vi "FP_Place FP on Point.vi"(8 "Error":errorcluster, 9 "FPSet":T1={"Menu Bar"=FALSE, "Position"=enum."MID-CTR", "Decoration index"=0, "border(px)"=-2, "Point"={"Left"=0, "Top"=0}}, 11 "VI Ref":refnum<vi>) -> (0 "Error Out":errorcluster, 3 "VI Ref Out":refnum<vi>)   [LabVIEW 2020]
doc: "sets up a fp to center of monitor 1 around largest decoration. shows scroll bars if developing and hides them if not."
uses:
  TypeDefs_Utility/Cluster_FP on Point Set.ctl
  TypeDefs_Utility/ENUM RB_Pos_Quadrant Position.ctl
  TypeDefs_Utility/Cluster_Top Left position.ctl
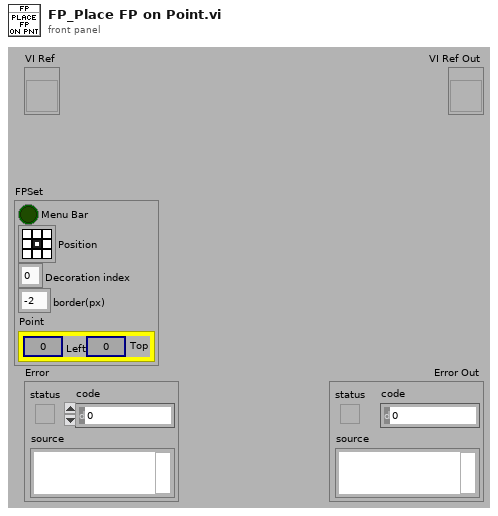
[diagram p1: front panel]
types:
  T1 = typedef "Cluster_FP on Point Set.ctl" = cluster{"Menu Bar":bool, "Position":T2, "Decoration index":i32, "border(px)":i32, "Point":T3}
  T2 = typedef "ENUM RB_Pos_Quadrant Position.ctl" = enum32{"LFT-TOP", "MID-TOP", "RGT-TOP", "LFT-CTR", "MID-CTR", "RGT-CTR", "LFT-BOT", "MID-BOT", "RGT-BOT"}
  T3 = typedef "Cluster_Top Left position.ctl" = cluster{"Left":i32, "Top":i32}
  T4 = enum32{"invalid app kind", "Development System", "Run Time System", "Student Edition", "Embedded LabVIEW", "Evaluation", "Custom"}
  T5 = enum32{"Invalid", "Standard", "Closed", "Hidden", "Minimized", "Maximized"}
  T6 = enum16{"Always On", "Always Off", "Off While Running"}
  T7 = typedef "LVRectTypeDef.ctl" = cluster{"Left":i16, "Top":i16, "Right":i16, "Bottom":i16}
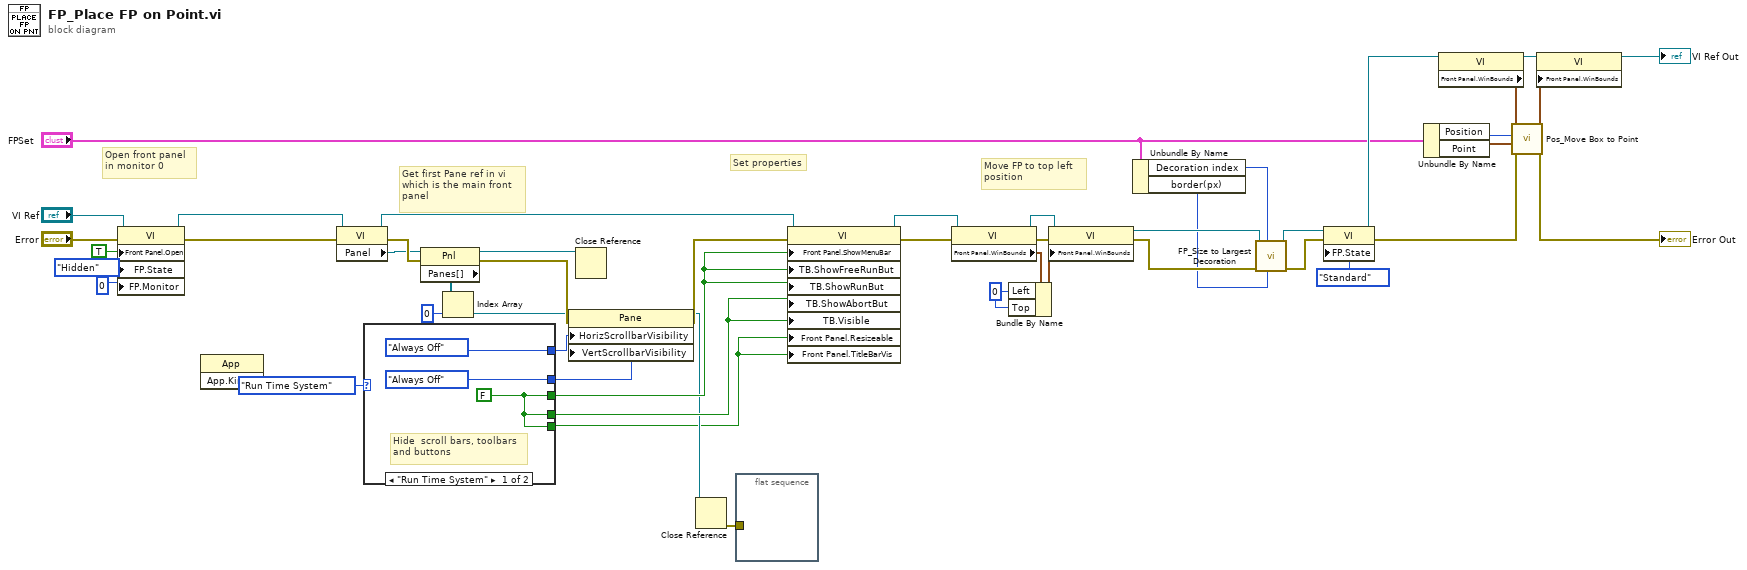
[diagram p0: block diagram]
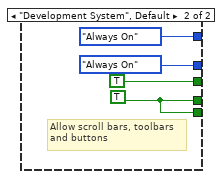
[diagram p2: hidden frame]
diagram:
  w24 = i16 0 ("left")
  # "Move FP to top left\nposition"
  # "Set properties"
  # "Get first Pane ref in vi\nwhich is the main front\npanel"
  # "Open front panel\nin monitor 0"
  n1 = property class="VI"(reference="VI Ref", error in="Error", "Front Panel.Open"=TRUE ("Front Panel Window:Open"), "FP.State"=T5."Hidden" ("Front Panel Window:State"), "FP.Monitor"=u16 0 ("Front Panel Window:Monitor")) -> (reference out=w19:refnum<vi>, error out=w20:errorcluster)
  n2 = property class="App" props=["App.Kind"]() -> ()  [unwired: 2 in, 3 out]
  n3 = property class="VI"(reference=w19, error in=w20) -> (reference out=w31:refnum<vi>, error out=w44:errorcluster, "Panel"=w40:refnum<vi>)
  n4 = case shown="\"Run Time System\"" T4."Run Time System" ("App.Kind") {
    tunnel: [T6."Always Off" ("Horizontal Scrollbar Visibility") T6."Always On" ("Horizontal Scrollbar Visibility")] -> w46
    tunnel: [w49 TRUE ("Front Panel Window:Show Menu Bar")] -> w11
    tunnel: [w49 w52] -> w33
    tunnel: [T6."Always Off" ("Horizontal Scrollbar Visibility") T6."Always On" ("Horizontal Scrollbar Visibility")] -> w32
    tunnel: [w49 w52] -> w1
    frame "Run Time System" {
      w49 = FALSE ("Front Panel Window:Show Menu Bar")
      # "Hide  scroll bars, toolbars\nand buttons"
    }
    frame "Development System", Default {
      w52 = TRUE ("Front Panel Window:Show Menu Bar")
      # "Allow scroll bars, toolbars\nand buttons"
    }
  }
  n5 = property class="Pnl"(reference=w40, error in=w44) -> (reference out=w34:refnum<vi>, error out=w43:errorcluster, "Panes[]"=w41:refnum<vi>[])
  n6 = Index Array(array=w41, index=0) -> (element=w42:refnum<vi>)
  n7 = property class="Pane"(reference=w42, error in=w43, "HorizScrollbarVisibility"=w32, "VertScrollbarVisibility"=w46) -> (reference out=w9:refnum<vi>, error out=w47:errorcluster)
  n8 = Close Reference(reference=w34) -> ()  [unwired: 1 in, 1 out]
  n9 = Close Reference(reference=w9) -> (error out=w18:errorcluster)  [unwired: 1 in]
  n10 = flat-sequence {
    tunnel: w18 -> [_]
    frame #0 {
    }
  }
  n11 = property class="VI"(reference=w31, error in=w47, "Front Panel.ShowMenuBar"=w11, "TB.ShowFreeRunBut"=w11, "TB.ShowRunBut"=w11, "TB.ShowAbortBut"=w33, "TB.Visible"=w33, "Front Panel.Resizeable"=w1, "Front Panel.TitleBarVis"=w1) -> (reference out=w30:refnum<vi>, error out=w28:errorcluster)
  n12 = property class="VI"(reference=w30, error in=w28) -> (reference out=w29:refnum<vi>, error out=w27:errorcluster, "Front Panel.WinBounds"=w26:T7)
  n13 = Bundle By Name(cluster=w26, "Left"=w24, "Top"=w24) -> (w25:T7)
  n14 = property class="VI"(reference=w29, error in=w27, "Front Panel.WinBounds"=w25) -> (reference out=w21:refnum<vi>, error out=w22:errorcluster)
  n15 = Unbundle By Name("FPSet") -> ("Decoration index"=w13:i32, "border(px)"=w12:i32)
  n16 = call "FP_Size to Largest Decoration.vi"("Border Spacing (2 Px)"=w12, "Decoration index"=w13, "Error"=w22, "VI Ref"=w21) -> ("Error Out"=w10:errorcluster, "VI Ref Out"=w23:refnum<vi>)  [unwired: 5 in, 1 out]
  n17 = property class="VI"(reference=w23, error in=w10, "FP.State"=T5."Standard" ("Front Panel Window:State")) -> (reference out=w15:refnum<vi>, error out=w8:errorcluster)
  n18 = Unbundle By Name("FPSet") -> ("Position"=w4:T2, "Point"=w5:T3)
  n19 = property class="VI"(reference=w15) -> (reference out=w14:refnum<vi>, "Front Panel.WinBounds"=w6:T7)  [unwired: 1 in, 1 out]
  n20 = call "Pos_Move Box to Point.vi"("Error"=w8, "Point"=w5, "Position"=w4, "Window"=w6) -> ("Error Out"=→"Error Out":errorcluster, "Window Out"=w17:T7)  [unwired: 6 in]
  n21 = property class="VI"(reference=w14, "Front Panel.WinBounds"=w17) -> (reference out=→"VI Ref Out":refnum<vi>)  [unwired: 1 in, 1 out]
